vi "Joystick breakout orig.vi"(0 "Joystick":T3) -> (4 "Axis":T2, 6 "Buttons":T1)   [LabVIEW 2014]
uses:
  <vilib>/Rock Robotics/WPI/Joystick/WPI_JoystickDevRef.ctl
  <vilib>/Rock Robotics/WPI/Joystick/WPI_JoystickDeviceEnum.ctl
panel:
  out "Button 10":bool
  out "Button 9":bool
  out "Button 8":bool
  out "Button 7":bool
  out "Button 6":bool
  out "Button 5":bool
  out "Button 4":bool
  out "Button 3":bool
  out "Button 2":bool
  out "Button 1":bool
  out "Axis 6":dbl
  out "Axis 5":dbl
  out "Axis 4":dbl
  out "Axis 3":dbl
  out "Axis 1":dbl
  out "Axis 2":dbl
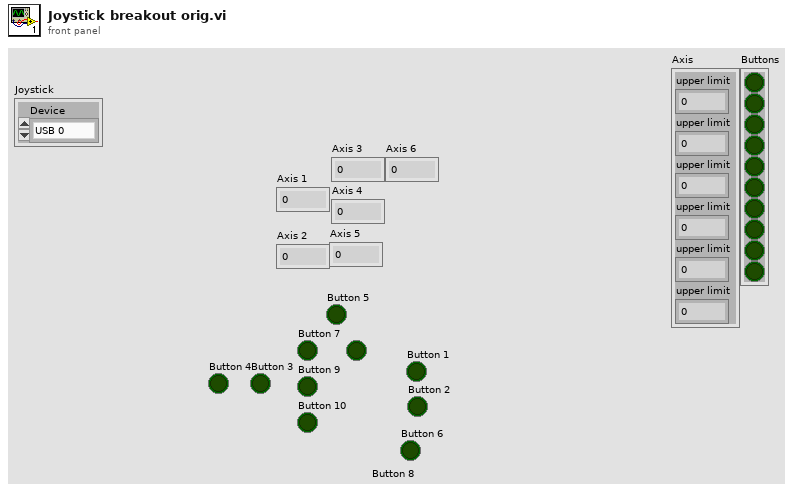
[diagram p1: front panel]
types:
  T1 = cluster{bool, bool, bool, bool, bool, bool, bool, bool, bool, bool}
  T2 = cluster{"upper limit":dbl, "upper limit":dbl, "upper limit":dbl, "upper limit":dbl, "upper limit":dbl, "upper limit":dbl}
  T3 = typedef "WPI_JoystickDevRef.ctl" = cluster{"Device":T4}
  T4 = typedef "WPI_JoystickDeviceEnum.ctl" = enum16{"USB 0", "USB 1", "USB 2", "USB 3", "USB 4", "USB 5"}
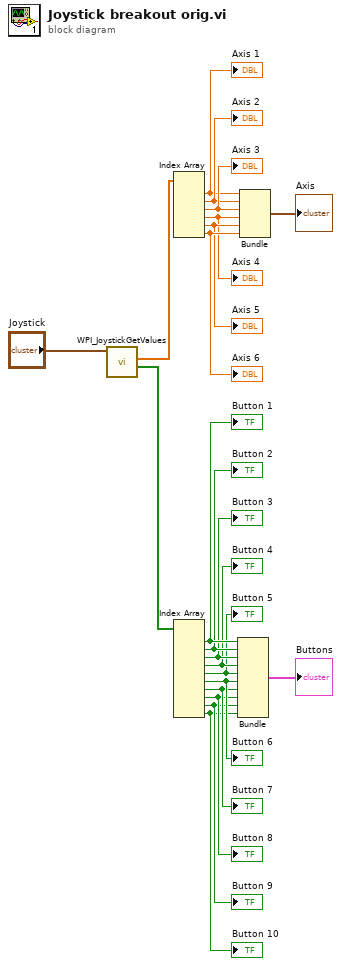
[diagram p0: block diagram]
diagram:
  n1 = call <vilib>:"WPI_JoystickGetValues.vi"("JoystickDevRef"="Joystick") -> ("Buttons"=w19:bool[], "Axes"=w20:dbl[])  [unwired: 6 in, 3 out]
  n2 = Index Array(array=w20) -> (element #1=w13:dbl, element #2=w14:dbl, element #3=w15:dbl, element #4=w16:dbl, element #5=w17:dbl, element #6=w18:dbl)  [unwired: 6 in]
  "Axis 2" <- w14
  "Axis 1" <- w13
  "Axis 3" <- w15
  "Axis 4" <- w16
  "Axis 5" <- w17
  "Axis 6" <- w18
  n3 = Index Array(array=w19) -> (element #1=w11:bool, element #2=w10:bool, element #3=w9:bool, element #4=w8:bool, element #5=w7:bool, element #6=w6:bool, element #7=w5:bool, element #8=w4:bool, element #9=w3:bool, element #10=w2:bool)  [unwired: 10 in]
  "Button 1" <- w11
  "Button 2" <- w10
  "Button 3" <- w9
  "Button 4" <- w8
  "Button 5" <- w7
  "Button 6" <- w6
  "Button 7" <- w5
  "Button 8" <- w4
  "Button 9" <- w3
  "Button 10" <- w2
  n4 = Bundle(w11, w10, w9, w8, w7, w6, w5, w4, w3, w2) -> (→"Buttons":T1)  [unwired: 1 in]
  n5 = Bundle("upper limit"=w13, "upper limit"=w14, "upper limit"=w15, "upper limit"=w16, "upper limit"=w17, "upper limit"=w18) -> (→"Axis":T2)  [unwired: 1 in]
